vi "Exam.vi"() -> ()   [LabVIEW 2018]
uses:
  6c2cfa1d-392a-4071-b661-849d02b3e7d9.vi
panel:
  out "확율 데이터 출력":dbl[](array[numeric])
  out "초기 데이터\n- 횟수":i32[](array[numeric])
  out "주사위값":dbl[](array[numeric])
  out "난수":dbl[](array[numeric])
  in  "주사위를 몇번 던지시겠습니까?":i32
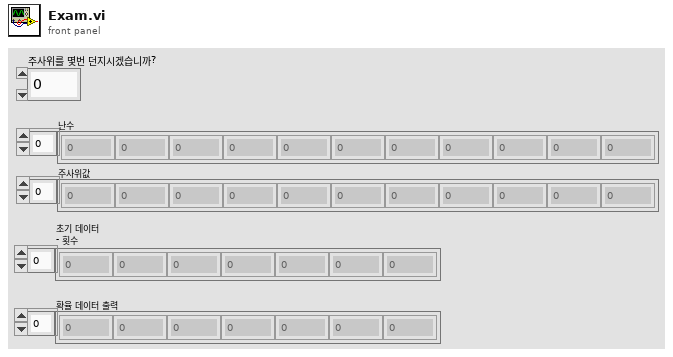
[diagram p1: front panel]
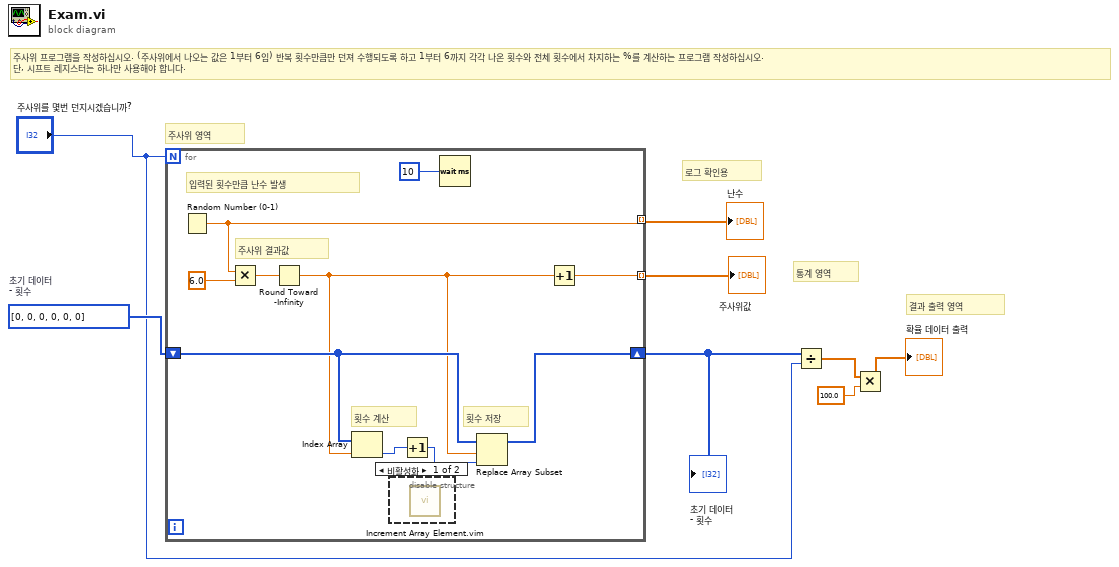
[diagram p0: block diagram]
diagram:
  w6 = i32[] [0, 0, 0, 0, 0, 0]  # 초기 데이터 - 횟수
  # "주사위 프로그램을 작성하십시오. (주사위에서 나오는 값은 1부터 6임) 반복 횟수만큼만 던져 수행되도록 하고 1부터 6까지 각각 나온 횟수와 전체 횟수에서 차지하는 %를 계산하는 프로그램 작성하십시오.\n단, 시프트 레지스터는 하나만 사용해야 합니다."
  # "로그 확인용"
  # "주사위 영역"
  # "통계 영역"
  # "결과 출력 영역"
  n1 = for {
    N: "주사위를 몇번 던지시겠습니까?" -> [_]
    tunnel: [w15] -> w8 mode=indexing
    tunnel: [w16] -> w7 mode=indexing
    shift-right: [w11] -> w5
    shift-left: w6 -> [w12]
    # "횟수 저장"
    # "횟수 계산"
    # "주사위 결과값"
    # "입력된 횟수만큼 난수 발생"
    n2 = Random Number (0-1)() -> (number: 0 to 1=w15:dbl)
    n3 = Multiply(x=w15, y=6.0) -> (x*y=w14:dbl)
    n4 = Round Toward -Infinity(1:w14) -> (0:w10:dbl)
    n5 = Index Array(array=w12, index=w10) -> (element=w13:i32)
    n6 = disable-structure shown="비활성화" {
      frame Disabled {
        n7 = call "Increment Array Element.vim"() -> ()  [unwired: 2 in, 1 out]
      }
      frame Enabled {
      }
    }
    n8 = Increment(x=w13) -> (x+1=w9:i32)
    n9 = Wait (ms)(milliseconds to wait=u32 10 ("대기 시간 (ms)")) -> ()  [unwired: 1 out]
    n10 = Replace Array Subset(array=w12, new element=w9, index=w10) -> (w11:i32[])
    n11 = Increment(x=w10) -> (x+1=w16:dbl)
  }
  "난수" <- w8
  "주사위값" <- w7
  "초기 데이터\n- 횟수" <- w5
  n12 = Divide(x=w5, y="주사위를 몇번 던지시겠습니까?") -> (x/y=w4:dbl[])
  n13 = Multiply(x=w4, y=100.0) -> (x*y=→"확율 데이터 출력":dbl[])
